vi "unusedWrite size.vi"(8 "error in (no error)":errorcluster, 10 "size":T1, 11 "Wire in":refnum<class "Terminal.lvclass">) -> (0 "error out":errorcluster, 3 "Wire out":refnum<class "Terminal.lvclass">)   [LabVIEW 2023]
uses:
  Terminal.lvclass/Terminal.ctl
  Terminal.lvclass
  <vilib>/Utility/miscctls.llb/LVBoundsTypeDef.ctl
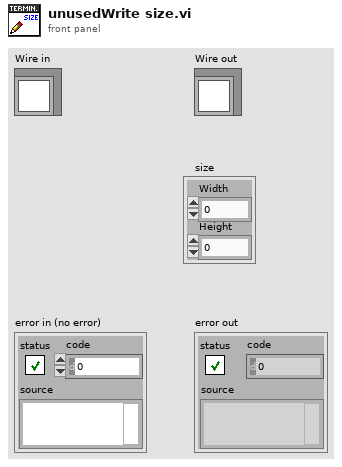
[diagram p1: front panel]
types:
  T1 = typedef "LVBoundsTypeDef.ctl" = cluster{"Width":u32, "Height":u32}
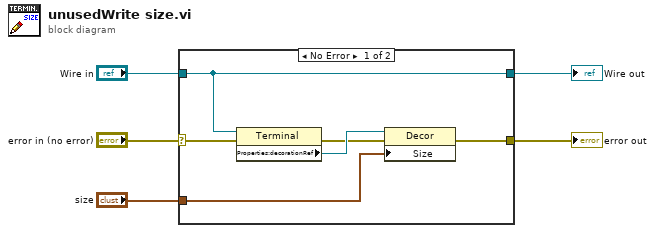
[diagram p0: block diagram]
diagram:
  n1 = case shown="No Error" "error in (no error)" {
    selector: "error in (no error)" -> [w8 w13]
    tunnel: [w7 w13] -> w4
    tunnel: [w11 w12] -> w2
    tunnel: "Wire in" -> [w11 w12]
    tunnel: "size" -> [w6 _]
    frame No Error {
      n2 = property class="Terminal"(reference=w11, error in=w8) -> (error out=w9:errorcluster, "Properties:decorationRef"=w10:refnum<vi>)  [unwired: 1 out]
      n3 = property class="Decor"(reference=w10, error in=w9, "Size"=w6) -> (error out=w7:errorcluster)  [unwired: 1 out]
    }
    frame Error {
    }
  }
  "error out" <- w4
  "Wire out" <- w2
